vi "Configure Output Limits.vi"(7 "Unit Address (1)":u8=1, 8 "error in (no error)":errorcluster, 9 "Output Limit Value (0)":sgl min=-1000 max=1000 format="%.1g", 10 "Enable Limit Type  (False: Low)":bool, 11 "VISA resource name":refnum<visa-resource-name>) -> (0 "error out":errorcluster, 3 "VISA resource name out":refnum<visa-resource-name>)   [LabVIEW 2014, in "Eurotherm 35xx Series.lvlib"]
doc: "This VI sets Output limits.\n\nDescription:\n\nMaximum-\nMaximum output power delivered by channels 1 and 2.\nBy reducing the high power limit, it is possible to reduce the rate of change of the process, however, care should be taken as reducing the power limit will reduce the controllers ability to react to disturbance.\n\nMinimum-\nMinimum (or maximum negative) output power delivered by channels 1 and 2.\nFor a 1 channel (heat only) algorithm this value will typically be set to 0%\nFor a 2 channel (heat/cool) algorithm this value will typically be set to -100%\nNote: the outputs in advanced controllers (e.g., 3504's) may also contain scaling parameters, these may be used to further restrict the power delivered."
uses:
  <instrlib>/Eurotherm 35xx Series/Eurotherm 35xx Series.lvlib
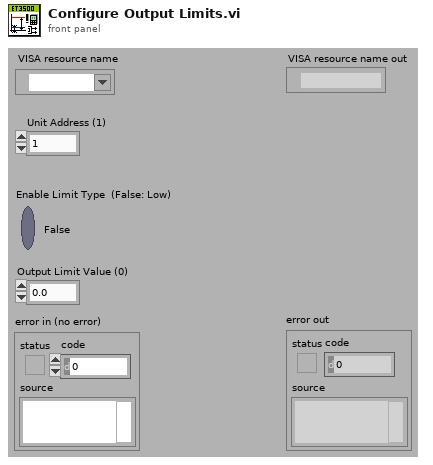
[diagram p1: front panel]
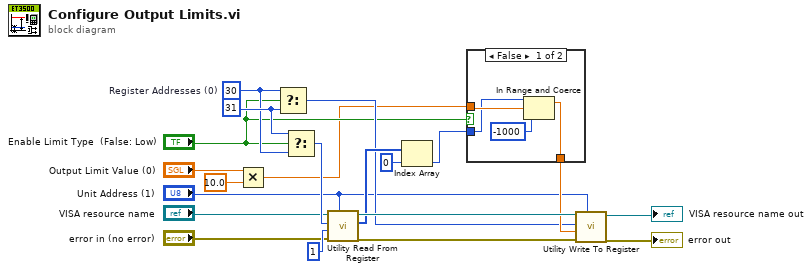
[diagram p0: block diagram]
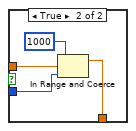
[diagram p2: hidden frame]
diagram:
  w17 = 31 ("Register Addresses (0)")
  w16 = 30  # Register Addresses (0)
  n1 = Multiply(x="Output Limit Value (0)", y=sgl 10.0) -> (x*y=w2:sgl)
  n2 = Select(t=w16, s="Enable Limit Type  (False: Low)", f=w17) -> (s? t:f=w10:i32)
  n3 = Select(t=w17, s="Enable Limit Type  (False: Low)", f=w16) -> (s? t:f=w15:i32)
  n4 = call <instrlib>:"Utility Read From Register.vi"("Unit Address (1)"="Unit Address (1)", "error in (no error)"="error in (no error)", "Num Of Reg (1)"=u16 1, "Register Address (0)"=w15, "VISA resource name"="VISA resource name") -> ("error out"=w19:errorcluster, "Data"=w14:i16[], "VISA resource name out"=w20:refnum<visa-resource-name>)  [unwired: 4 in]
  n5 = Index Array(array=w14, index=0) -> (element=w12:i16)
  n6 = case shown="False" "Enable Limit Type  (False: Low)" {
    tunnel: w12 -> [w22 w27]
    tunnel: w2 -> [w24 w26]
    tunnel: [w21 w25] -> w11
    frame False {
      n7 = In Range and Coerce(upper limit=w22, x=w24, lower limit=-1000 ("upper limit")) -> (coerced(x)=w21:sgl)  [unwired: 1 out]
    }
    frame True {
      n8 = In Range and Coerce(upper limit=1000, x=w26, lower limit=w27) -> (coerced(x)=w25:sgl)  [unwired: 1 out]
    }
  }
  n9 = call <instrlib>:"Utility Write To Register.vi"("Unit Address (1)"="Unit Address (1)", "error in (no error)"=w19, "Data (0)"=w11, "Register Address (0)"=w10, "VISA resource name"=w20) -> ("error out"=→"error out":errorcluster, "VISA resource name out"=→"VISA resource name out":refnum<visa-resource-name>)  [unwired: 5 in]
